vi "test-ElevatorSim-stability.vi"() -> (3 "Test Passed":bool)   [LabVIEW 2019]
uses:
  <vilib>/Rock Robotics/WPI/ThirdParty/JAS_Junk/TrajLib/DCMOTOR.CTL
  <vilib>/Rock Robotics/WPI/ThirdParty/JAS_Junk/TrajLib/ELEVATOR_SIM.ctl
  <vilib>/Rock Robotics/WPI/ThirdParty/JAS_Junk/TrajLib/LINEAR_SYSTEM_SIM.ctl
  <vilib>/Rock Robotics/WPI/ThirdParty/JAS_Junk/TrajLib/LINEAR_SYSTEM.ctl
  <vilib>/Analysis/Matrix/Datatypes/RealMatrix.ctl
  <vilib>/Rock Robotics/WPI/ThirdParty/JAS_Junk/TrajLib/MatBuilder_Create.vi
  <vilib>/Rock Robotics/WPI/ThirdParty/JAS_Junk/TrajLib/DCMotor_New.vi
  <vilib>/Rock Robotics/WPI/ThirdParty/JAS_Junk/TrajLib/Units_RotationsPerMinuteToRadiansPerSecond.vi
  <vilib>/Rock Robotics/WPI/ThirdParty/JAS_Junk/TrajLib/Discretization_DiscretizeAB.vi
  <vilib>/Analysis/baseanly.llb/A x B.vi
  <vilib>/Analysis/baseanly.llb/Real A x B.vi
  <vilib>/Rock Robotics/WPI/ThirdParty/JAS_Junk/TrajLib/MatrixHelper_CoerceSize.vi
  <vilib>/Rock Robotics/WPI/ThirdParty/JAS_Junk/TrajLib/Matrix_Exp.vi
  <vilib>/Rock Robotics/WPI/ThirdParty/JAS_Junk/TrajLib/Matrix_AssignBlock.vi
  <vilib>/Rock Robotics/WPI/ThirdParty/JAS_Junk/TrajLib/Matrix_ExtractFrom.vi
  <vilib>/Analysis/7linalg.llb/Matrix Exp.vi
  <vilib>/Analysis/7linalg.llb/Real Matrix Exp.vi
  <vilib>/Analysis/Matrix/Numeric/Multiply/Multiply.vi
  <vilib>/Analysis/Matrix/Numeric/Multiply/Multiply - RM,R.vi
  <vilib>/Analysis/Matrix/Numeric/Add/Add.vi
  <vilib>/Analysis/Matrix/Numeric/Add/Add - RM,RM.vi
  <vilib>/Rock Robotics/WPI/ThirdParty/JAS_Junk/TrajLib/Trajectory_Library.lvlib
  <vilib>/Analysis/Matrix/NI_Matrix.lvlib
panel:
  in  "Tab Control":enum32{"Page 2", "Page 6", "Page 7"}(tab)
  out "Elevator Motor":T1 {"Jr_KgM2" format="%13.5p"; "L_H" format="%13.5p"; "Kt_NMPerAmp" format="%13.5p"; "KvINV_RadPerSecPerVolt" format="%13.5p"; "R_Ohms" format="%13.5p"; "FreeSpeed_RadPerSec" format="%13.5p"; "FreeCurrent_Amps" format="%13.5p"; "StallCurrent_Amps" format="%13.5p"; "StallTorque_NM" format="%13.5p"; "nominalVoltage_Volts" format="%13.5p"}
  out "Elevator Simulaation":T2 {"GearBox"."Jr_KgM2" format="%13.5p"; "GearBox"."L_H" format="%13.5p"; "GearBox"."Kt_NMPerAmp" format="%13.5p"; "GearBox"."KvINV_RadPerSecPerVolt" format="%13.5p"; "GearBox"."R_Ohms" format="%13.5p"; "GearBox"."FreeSpeed_RadPerSec" format="%13.5p"; "GearBox"."FreeCurrent_Amps" format="%13.5p"; "GearBox"."StallCurrent_Amps" format="%13.5p"; "GearBox"."StallTorque_NM" format="%13.5p"; "GearBox"."nominalVoltage_Volts" format="%13.5p"}
  out "Velocity":cluster{"Voltage":dbl}(graph)
  out "PV Chart":cluster{dbl}(graph)
  out "At Top":bool
  out "At Bottom":bool
  out "Size Coerced":bool
  out "Alt Position Meters":dbl
  out "Position_Meters":dbl
  out "ApproxEquals":bool
  # "<States, 1>"
  # "<Outputs, 1>"
  # "<Inputs, 1>"
  # "<Outputs, 1>"
  # "<States,States>"
  # "<States,Inputs>"
  # "<Outputs,States>"
  # "<Outputs,Inputs>"
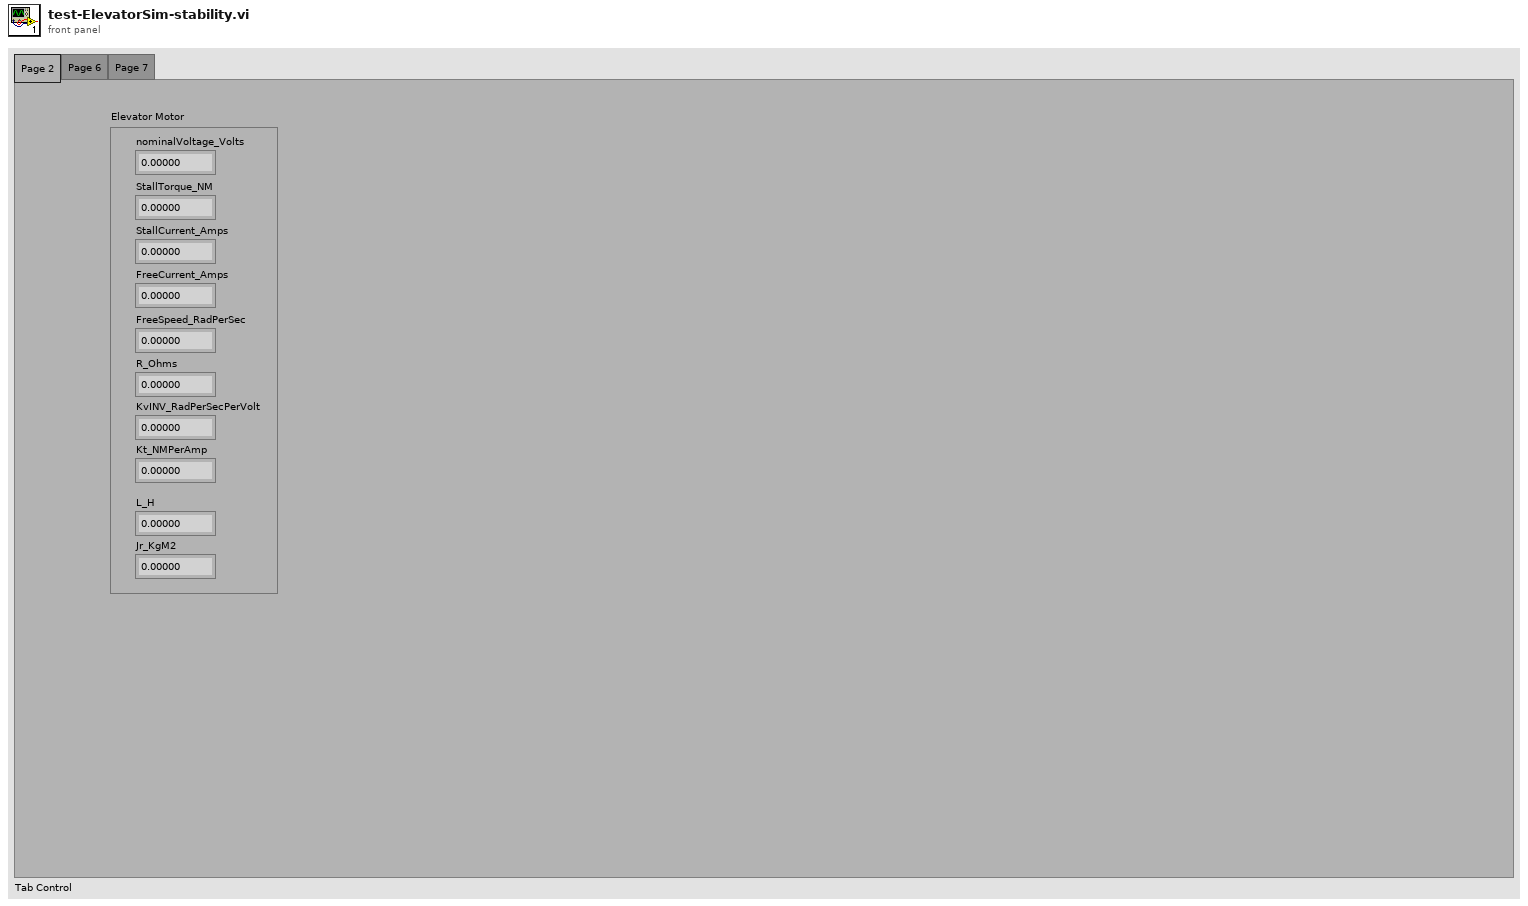
[diagram p1: front panel]
types:
  T1 = typedef "Trajectory_Library.lvlib/DCMOTOR.CTL" = cluster{"nominalVoltage_Volts":dbl, "StallTorque_NM":dbl, "StallCurrent_Amps":dbl, "FreeCurrent_Amps":dbl, "FreeSpeed_RadPerSec":dbl, "R_Ohms":dbl, "KvINV_RadPerSecPerVolt":dbl, "Kt_NMPerAmp":dbl, "L_H":dbl, "Jr_KgM2":dbl}
  T2 = typedef "Trajectory_Library.lvlib/ELEVATOR_SIM.ctl" = cluster{"LinearSystemSim":T3, "GearBox":T1, "Gearing":dbl, "DrumRadius_M":dbl, "MinHeight_M":dbl, "MaxHeight_M":dbl, "CarriageMass_Kg":dbl}
  T3 = typedef "Trajectory_Library.lvlib/LINEAR_SYSTEM_SIM.ctl" = cluster{"m_Plant":T4, "m_X":T5, "m_Y":T5, "m_U":T5, "MeasureStdDev":T5}
  T4 = typedef "Trajectory_Library.lvlib/LINEAR_SYSTEM.ctl" = cluster{"m_A":T5, "m_B":T5, "m_C":T5, "m_D":T5, "States":i32, "Inputs":i32, "Outputs":i32}
  T5 = typedef "NI_Matrix.lvlib/RealMatrix.ctl" = dbl[][]
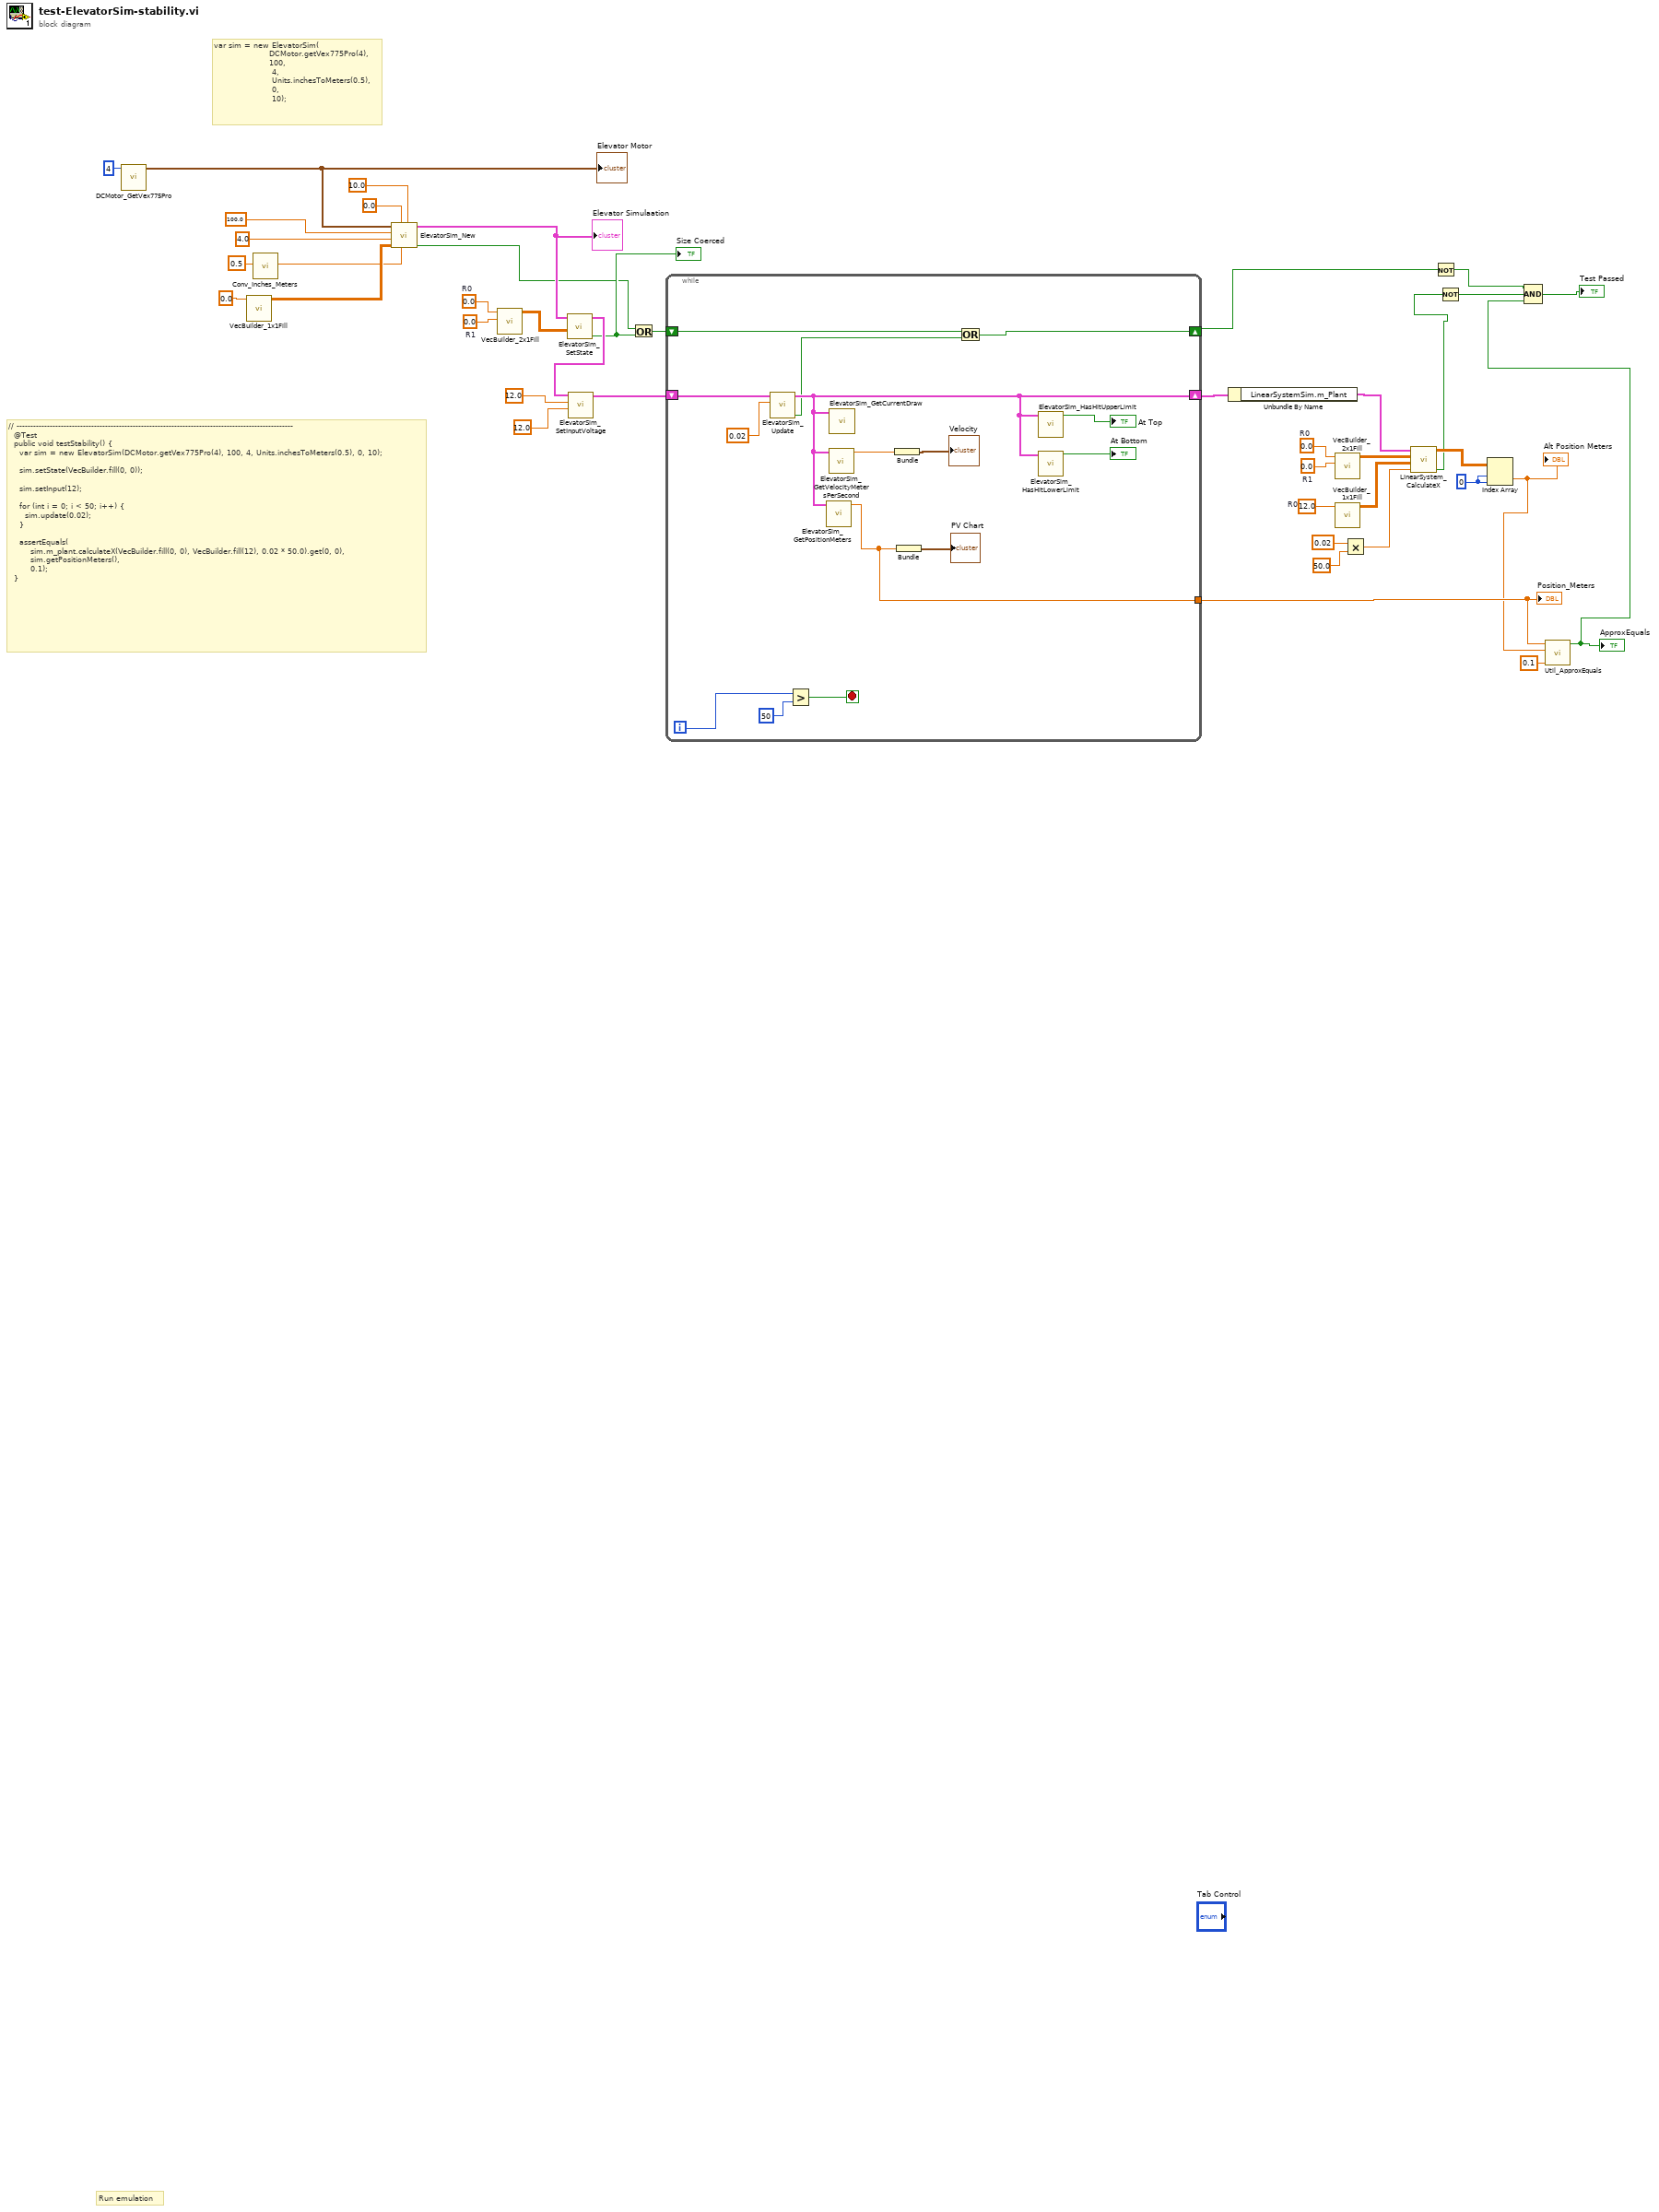
[diagram p0: block diagram]
diagram:
  w13 = 0 ("index (row)")
  w20 = 12.0  # R0
  w22 = 0.0  # R1
  w21 = 0.0  # R0
  w27 = 0.0  # R1
  w26 = 0.0  # R0
  # "// ----------------------------------------------------------------------------------------------------\n  @Test\n  public void testStability() {\n    var sim = new ElevatorSim(DCMotor.getVex775Pro(4), 100, 4, Units.inchesToMeters(0.5), 0, 10);\n\n    sim.setState(VecBuilder.fill(0, 0));\n\n    sim.setInput(12);\n\n    for (int i = 0; i < 50; i++) {\n      sim.update(0.02);\n    }\n\n    assertEquals(\n        sim.m_plant.calculateX(VecBuilder.fill(0, 0), VecBuilder.fill(12), 0.02 * 50.0).get(0, 0),\n        sim.getPositionMeters(),\n        0.1);\n  }"
  # "var sim = new ElevatorSim(\n                    DCMotor.getVex775Pro(4), \n                    100, \n                     4, \n                     Units.inchesToMeters(0.5), \n                     0, \n                     10);"
  # "Run emulation"
  n1 = call <vilib>:"DCMotor_GetVex775Pro.vi"("Num Motors"=4) -> ("DCMOTOR"=w35:T1)  [unwired: 10 in]
  "Elevator Motor" <- w35
  n2 = call <vilib>:"VecBuilder_1x1Fill.vi"("R0_C0"=0.0) -> ("output matrix"=w39:T5)  [unwired: 10 in]
  n3 = call <vilib>:"Conv_Inches_Meters.vi"("INCH"=0.5) -> ("Meters"=w33:dbl)  [unwired: 10 in]
  n4 = call <vilib>:"ElevatorSim_New.vi"("MaxHeight_Meters"=10.0, "DrumRadius_Meters"=w33, "MinHeight_Meters"=0.0, "MeasurementStdDev"=w39, "CarriageMass_Kg"=4.0 ("massKg"), "Gearing"=100.0 ("G"), "GearBox"=w35) -> ("Error"=w3:bool, "ElevatorSim"=w29:T2)  [unwired: 3 in]
  "Elevator Simulaation" <- w29
  n5 = call <vilib>:"VecBuilder_2x1Fill.vi"("R1"=w27, "R0"=w26) -> ("output matrix"=w25:T5)  [unwired: 9 in]
  n6 = call <vilib>:"ElevatorSim_SetState.vi"("System State"=w25, "in ElevatorSim"=w29) -> ("Size Coerced"=w4:bool, "out ElevatorSim"=w28:T2)  [unwired: 8 in]
  "Size Coerced" <- w4
  n7 = call <vilib>:"ElevatorSim_SetInputVoltage.vi"("Battery_Volts"=12.0, "Input_Voltage"=12.0, "in ElevatorSim"=w28) -> ("out ElevatorSim"=w30:T2)  [unwired: 8 in]
  n8 = Or(x=w3, y=w4) -> (x .or. y?=w5:bool)
  n9 = while {
    shift-right: [w51] -> w24
    shift-left: w30 -> [w53]
    tunnel: [w46] -> w12
    shift-right: [w43] -> w2
    shift-left: w5 -> [w44]
    i -> [w49]
    stop <- w47 stop-if-true
    n10 = call <vilib>:"ElevatorSim_Update.vi"("dT_Seconds"=0.02, "in ElevatorSim"=w53) -> ("Error"=w45:bool, "out ElevatorSim"=w51:T2)  [unwired: 8 in]
    n11 = Greater?(x=w49, y=50) -> (0:w47:bool)
    n12 = call <vilib>:"ElevatorSim_GetPositionMeters.vi"("ElevatorSim"=w51) -> ("Position_Meters"=w46:dbl)  [unwired: 10 in]
    n13 = call <vilib>:"ElevatorSim_GetVelocityMetersPerSecond.vi"("ElevatorSim"=w51) -> ("Velocity_MetersPerSec"=w50:dbl)  [unwired: 10 in]
    n14 = call <vilib>:"ElevatorSim_GetCurrentDraw.vi"("ElevatorSim"=w51) -> ()  [unwired: 10 in, 1 out]
    n15 = Bundle("Velocity_MetersPerSec"=w50) -> (→"Velocity":cluster{"Velocity_MetersPerSec":dbl})  [unwired: 1 in]
    n16 = Bundle("Position_Meters"=w46) -> (→"PV Chart":cluster{"Position_Meters":dbl})  [unwired: 1 in]
    n17 = Or(x=w44, y=w45) -> (x .or. y?=w43:bool)
    n18 = call <vilib>:"ElevatorSim_HasHitUpperLimit.vi"("ElevatorSim"=w51) -> ("At HIgh LImit"=→"At Top":bool)  [unwired: 10 in]
    n19 = call <vilib>:"ElevatorSim_HasHitLowerLimit.vi"("ElevatorSim"=w51) -> ("AtLowLimit"=→"At Bottom":bool)  [unwired: 10 in]
  }
  "Position_Meters" <- w12
  n20 = Unbundle By Name(w24) -> ("LinearSystemSim.m_Plant"=w23:T4)
  n21 = call <vilib>:"VecBuilder_2x1Fill.vi"("R1"=w22, "R0"=w21) -> ("output matrix"=w19:T5)  [unwired: 9 in]
  n22 = call <vilib>:"VecBuilder_1x1Fill.vi"("R0_C0"=w20) -> ("output matrix"=w18:T5)  [unwired: 10 in]
  n23 = Multiply(x=0.02, y=50.0) -> (x*y=w15:dbl)
  n24 = call <vilib>:"LinearSystem_CalculateX.vi"("dT_Seconds"=w15, "ClampedU"=w18, "X"=w19, "Linearsystem"=w23) -> ("Error"=w7:bool, "outX"=w14:T5)  [unwired: 6 in]
  n25 = Not(x=w2) -> (.not. x?=w1:bool)
  n26 = Not(x=w7) -> (.not. x?=w6:bool)
  n27 = Index Array(array=w14, index (row)=w13, index (col)=w13) -> (element=w11:dbl)
  "Alt Position Meters" <- w11
  n28 = call <vilib>:"Util_ApproxEquals.vi"("Tolerance"=0.1, "Value 2"=w11, "Value 1"=w12) -> ("ApproxEquals"=w8:bool)  [unwired: 8 in]
  "ApproxEquals" <- w8
  n29 = Compound Arithmetic op=AND(w1, w6, w8) -> (→"Test Passed":bool)
